vi "chat_ui_tester.vi"() -> ()   [LabVIEW 2020]
uses:
  src/user_interfaces/simple_html_chat_ui/simple_html_chat_ui.lvclass
panel:
  in  "stop":bool
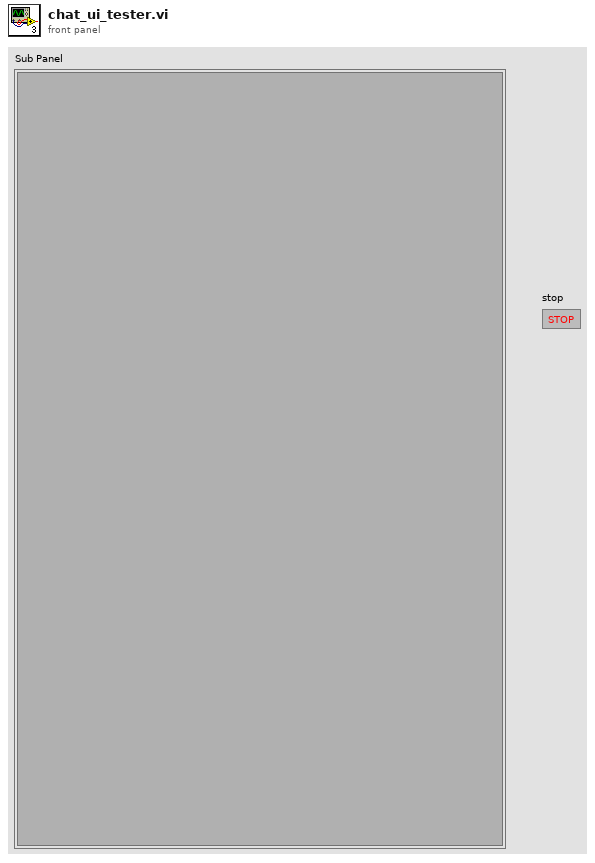
[diagram p1: front panel]
types:
  T1 = typedef "simple_html_chat_ui.lvclass/web_events.ctl" = cluster{"User prompt":refnum<user-event>, "Clear history":refnum<user-event>}
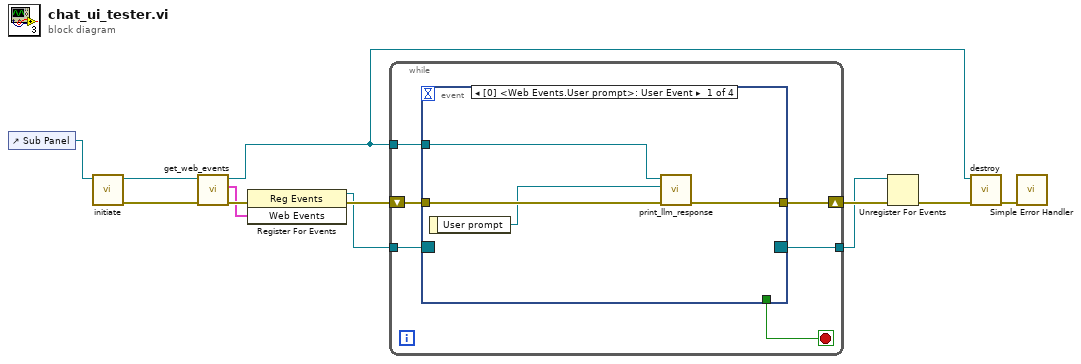
[diagram p0: block diagram]
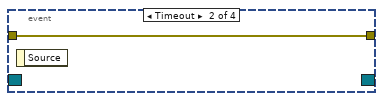
[diagram p2: hidden frame]
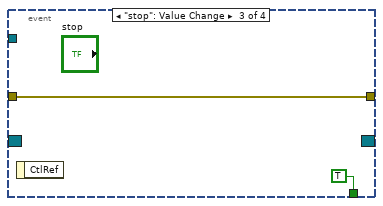
[diagram p3: hidden frame]
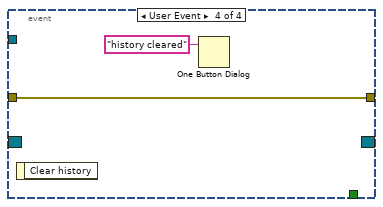
[diagram p4: hidden frame]
diagram:
  n1 = control-ref of="Sub Panel"() -> (w12:refnum<vi>)
  n2 = call "initiate.vi"("Sub Panel"=w12) -> ("error out"=w11:errorcluster, "simple_html_chat_ui out"=w10:refnum<class "simple_html_chat_ui.lvclass">)  [unwired: 9 in]
  n3 = call "get_web_events.vi"("error in (no error)"=w11, "simple_html_chat_ui in"=w10) -> ("error out"=w9:errorcluster, "Web Events"=w8:T1, "simple_html_chat_ui out"=w2:refnum<class "simple_html_chat_ui.lvclass">)  [unwired: 7 in]
  n4 = register-events(error in=w9, w8) -> (reference out=w6:refnum<event-registration>, error out=w7:errorcluster)  [unwired: 1 in]
  n5 = while {
    tunnel: w6 -> [w18]
    tunnel: w2 -> [w16]
    shift-right: [w15] -> w5
    shift-left: w7 -> [w17]
    tunnel: [w14] -> w4
    stop <- w13 stop-if-true
    n6 = event shown="[0] <Web Events.User prompt>: User Event" {
      selector: w18 -> [_ _ _ _]
      dyn-events: [_ _ _ _] -> w14
      timeout: _ -> [_ _ _ _]
      tunnel: w17 -> [w22 w23 w25 w27]
      tunnel: w16 -> [w21 _ _ _]
      tunnel: [w20 w23 w25 w27] -> w15
      tunnel: [_ _ TRUE _] -> w13
      event User Event {
        n7 = event-data() -> ("User prompt"=w19:refnum<class "abstract_message_base.lvclass">)  [unwired: 1 in]
        n8 = call "print_llm_response.vi"("error in (no error)"=w22, "llm_response"=w19, "simple_html_chat_ui in"=w21) -> ("error out"=w20:errorcluster)  [unwired: 7 in, 1 out]
      }
      event Timeout {
        n9 = event-data() -> ()  [unwired: 1 in, 1 out]
      }
      event "stop": Value Change {
        n10 = event-data() -> ()  [unwired: 1 in, 1 out]
      }
      event User Event {
        n11 = event-data() -> ()  [unwired: 1 in, 1 out]
        n12 = One Button Dialog(message="history cleared") -> ()  [unwired: 1 in, 1 out]
      }
    }
  }
  n13 = Unregister For Events(event registration refnum=w4, error in=w5) -> (error out=w3:errorcluster)
  n14 = call "destroy.vi"("error in (no error)"=w3, "simple_html_chat_ui in"=w2) -> ("error out"=w1:errorcluster)  [unwired: 8 in, 1 out]
  n15 = call <vilib>:"Simple Error Handler.vi"("error in (no error)"=w1) -> ()  [unwired: 4 in, 5 out]
